vi "Constants.vi"() -> ()   [LabVIEW 2023, in "HPS-17000 Custom Device Shared.lvlib"]
doc: "Use this Global VI to access the GUIDs assigned to the page resources of the Custom Device."
uses:
  HPS-17000 Custom Device Shared.lvlib
panel:
  in  "Tab Control":enum32{"GUIDs", "Constants", "Properties"}(tab)
  in  "HPS-17000 Custom Device":string="04f632e1-4a14-4b46-b342-fa2f795eb632"
  in  "Compiled.Settings":string="Compiled.Settings"
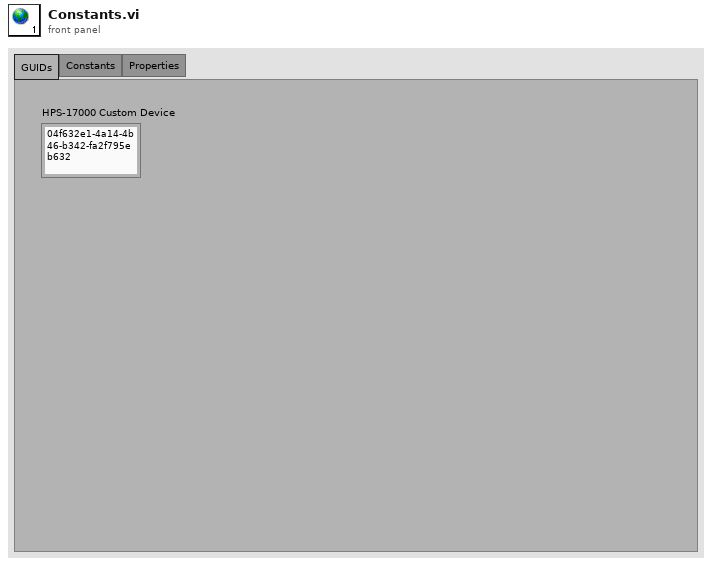
[diagram p1: front panel]
diagram:
